vi "Aula 2avi.vi"() -> ()   [LabVIEW 2024]
panel:
  in  "Numeric":dbl
  out "Iterações 2":dbl
  in  "Temperatura ºF 2":dbl(slide) scale=0.0..273.0
  out "Temperatura ºC 3":dbl(slide) scale=0.0..100.0
  out "Temperatura ºC 2":dbl
  in  "stop 2":bool
  in  "Boolean 2":bool
  out "Iterações":dbl
  out "Temperatura ºC":dbl(slide) scale=0.0..100.0
  out "Temperatura ºC":dbl
  in  "Temperatura ºF":dbl(slide) scale=0.0..273.0
  in  "stop":bool
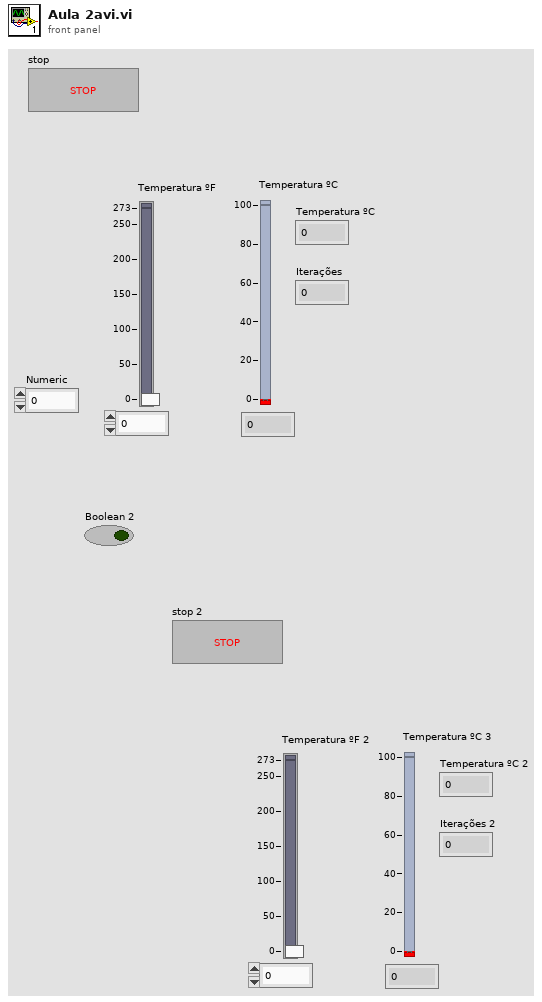
[diagram p1: front panel]
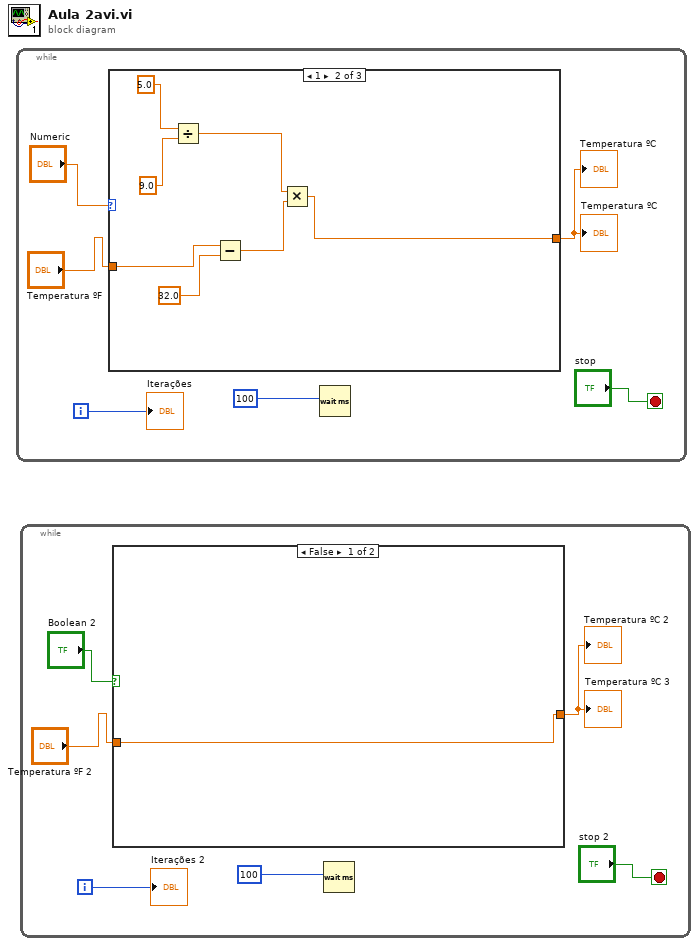
[diagram p0: block diagram]
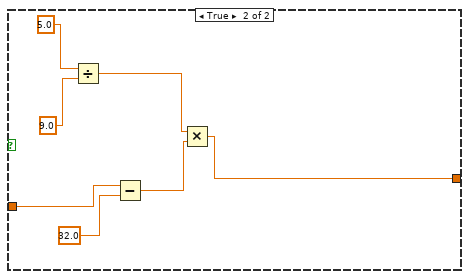
[diagram p2: hidden frame]
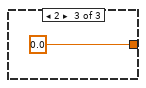
[diagram p4: hidden frame]
diagram:
  n1 = while {
    i -> [w6]
    stop <- "stop" stop-if-true
    n2 = case shown="1" "Numeric" {
      tunnel: "Temperatura ºF" -> [w7 w9 _]
      tunnel: [w7 w8 0.0 ("Temperatura ºF")] -> w4
      frame 0, Default {
      }
      frame 1 {
        n3 = Divide(x=5.0, y=9.0) -> (x/y=w11:dbl)
        n4 = Subtract(x=w9, y=32.0) -> (x-y=w10:dbl)
        n5 = Multiply(x=w11, y=w10) -> (x*y=w8:dbl)
      }
      frame 2 {
      }
    }
    "Temperatura ºC" <- w4
    "Temperatura ºC" <- w4
    n6 = Wait (ms)(milliseconds to wait=u32 100) -> ()  [unwired: 1 out]
    "Iterações" <- w6
  }
  n7 = while {
    i -> [w21]
    stop <- "stop 2" stop-if-true
    n8 = case shown="False" "Boolean 2" {
      tunnel: "Temperatura ºF 2" -> [w22 w24]
      tunnel: [w22 w23] -> w19
      frame False {
      }
      frame True {
        n9 = Divide(x=5.0, y=9.0) -> (x/y=w26:dbl)
        n10 = Subtract(x=w24, y=32.0) -> (x-y=w25:dbl)
        n11 = Multiply(x=w26, y=w25) -> (x*y=w23:dbl)
      }
    }
    "Temperatura ºC 3" <- w19
    "Temperatura ºC 2" <- w19
    n12 = Wait (ms)(milliseconds to wait=u32 100) -> ()  [unwired: 1 out]
    "Iterações 2" <- w21
  }
